vi "Popup_OptoStim.vi"(8 "에러 입력(에러 없음)":errorcluster, 9 "[OptoStim]Changed?":bool, 10 "Caller VI Reference":refnum<vi>, 11 "Parameters for Optic stimulation (NI)":T1) -> (0 "에러 출력":errorcluster, 3 "Parameters for Optic stimulation (OUT)":T1)   [LabVIEW 2017]
uses:
  Class, Controls/Parameters for Optic Stimulation.ctl
panel:
  in  "Parameters for Optic stimulation":T1={"Begin (sec)"="0.51232", "Frequency (Hz)"="10", "Number of Epoch"="12", "Time window (ms)"="30"}
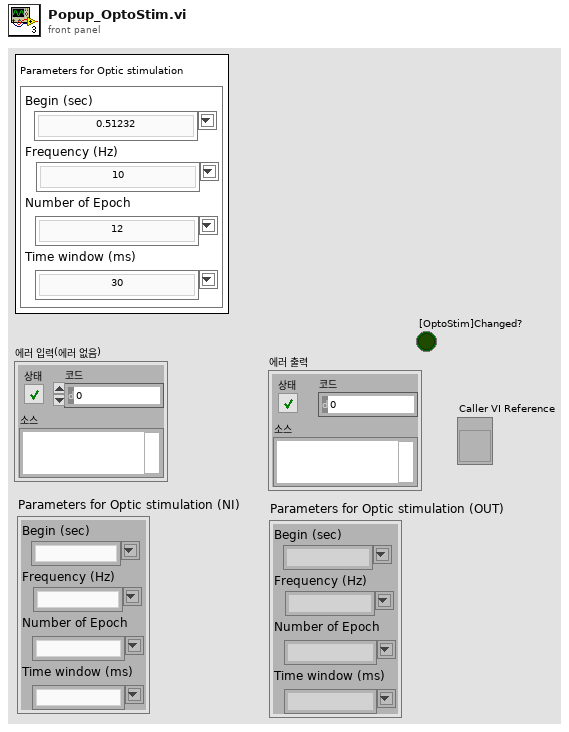
[diagram p1: front panel]
types:
  T1 = typedef "Parameters for Optic Stimulation.ctl" = cluster{"Begin (sec)":string, "Frequency (Hz)":string, "Number of Epoch":string, "Time window (ms)":string}
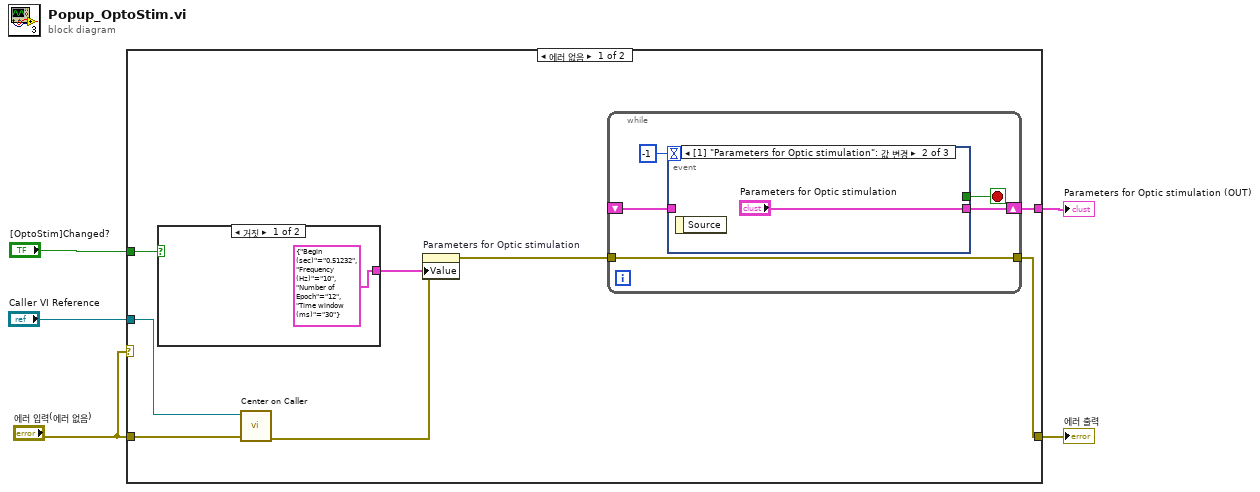
[diagram p0: block diagram]
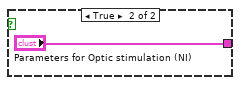
[diagram p2: hidden frame]
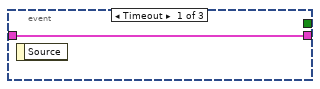
[diagram p3: hidden frame]
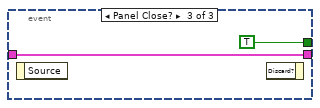
[diagram p4: hidden frame]
diagram:
  n1 = case shown="에러 없음" "에러 입력(에러 없음)" {
    tunnel: [w13 _] -> w5
    tunnel: "에러 입력(에러 없음)" -> [w8 w25]
    tunnel: [w10 w25] -> w4
    tunnel: "[OptoStim]Changed?" -> [w9 _]
    tunnel: "Caller VI Reference" -> [w6 _]
    frame No Error {
      n2 = case shown="거짓" w9 {
        tunnel: [T1 {"Begin (sec)"="0.51232", "Frequency (Hz)"="10", "Number of Epoch"="12", "Time window (ms)"="30"} ("Parameters for Optic stimulation 2") "Parameters for Optic stimulation (NI)"] -> w12
        frame False {
        }
        frame True {
        }
      }
      n3 = call <userlib>:"Center on Caller.vi"("에러 입력(에러 없음)"=w8, "Caller VI Reference"=w6) -> ("에러 출력"=w7:errorcluster)  [unwired: 9 in]
      n4 = property on="Parameters for Optic stimulation" class="Clust (엄격한)"(error in=w7, "Value"=w12) -> (error out=w11:errorcluster)  [unwired: 1 in, 1 out]
      n5 = while {
        shift-right: [w19] -> w13
        shift-left: _ -> [w20]
        tunnel: w11 -> [w16]
        tunnel: [w16] -> w10
        stop <- w18 stop-if-true
        n6 = event shown="[1] \"Parameters for Optic stimulation\": 값 변경" {
          selector: _ -> [_ _ _]
          dyn-events: _ -> [_ _ _]
          timeout: -1 -> [_ _ _]
          tunnel: w20 -> [w21 _ w23]
          tunnel: [w21 "Parameters for Optic stimulation" w23] -> w19
          tunnel: [_ _ TRUE] -> w18
          event Timeout {
            n7 = event-data() -> ()  [unwired: 1 in, 1 out]
          }
          event Value Change {
            n8 = event-data() -> ()  [unwired: 1 in, 1 out]
          }
          event Panel Close? {
            n9 = event-data() -> ()  [unwired: 1 in, 1 out]
            n10 = event-data() -> ()  [unwired: 2 in, 1 out]
          }
        }
      }
    }
    frame Error {
    }
  }
  "Parameters for Optic stimulation (OUT)" <- w5
  "에러 출력" <- w4
